vi "Compensate direction motor.vi"() -> ()   [LabVIEW 2011]
panel:
  out "DSO1072B":refnum<visa-resource-name>="USB0::0x0957::0x0588::CN55040431::INSTR"
  out "MUX RELAY":refnum<visa-resource-name>
  out "PWIDTH":dbl format="%#_6f"
  out "MAX AMP":dbl format="%#_6f"
  out "read buffer":string
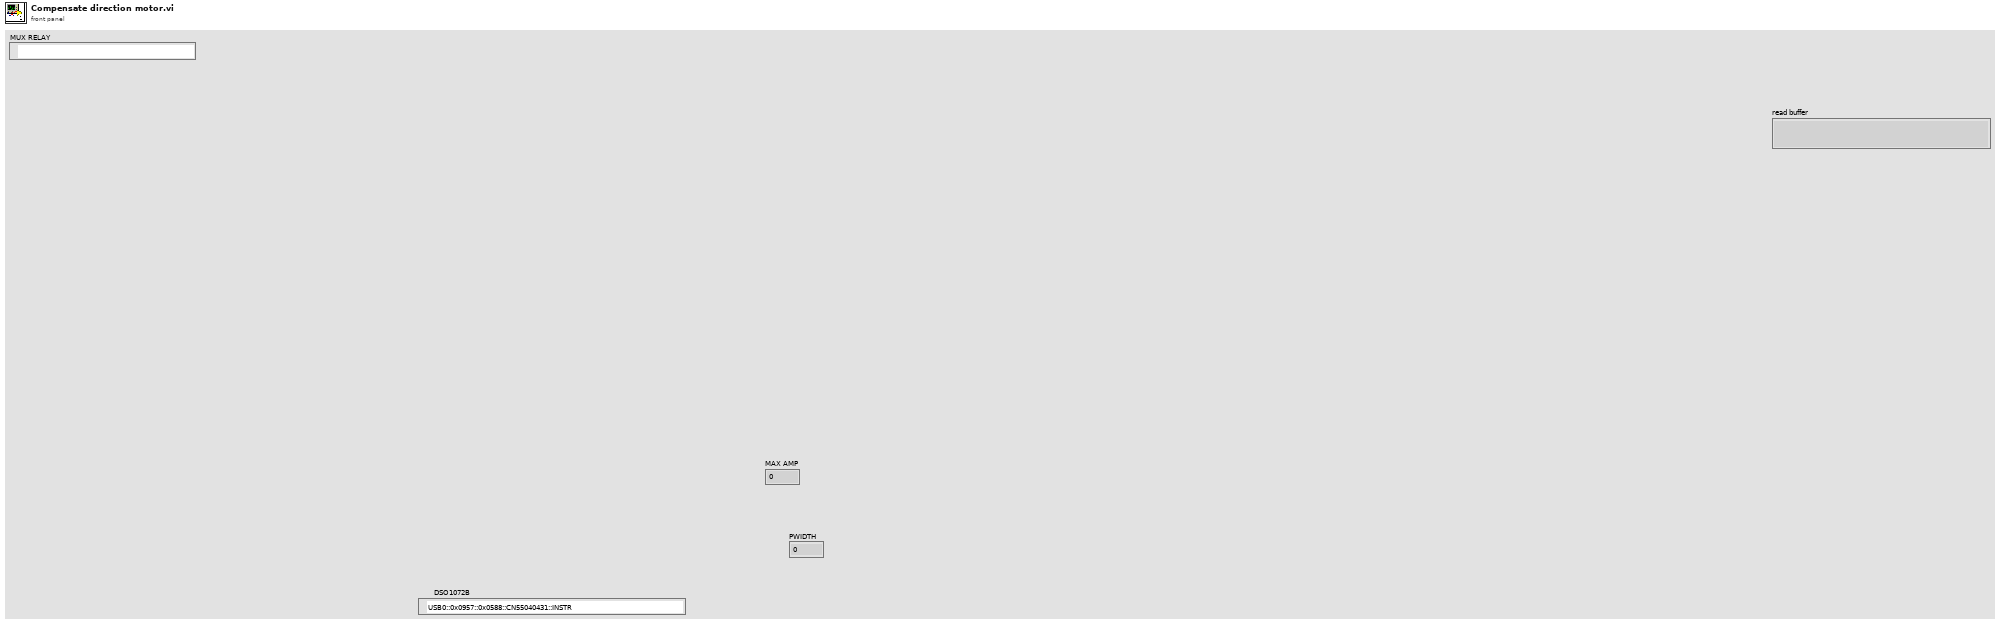
[diagram p1: front panel]
types:
  T1 = enum32{"Set Relay", "Append Relay", "Clear Relay", "Manual Cmd"}
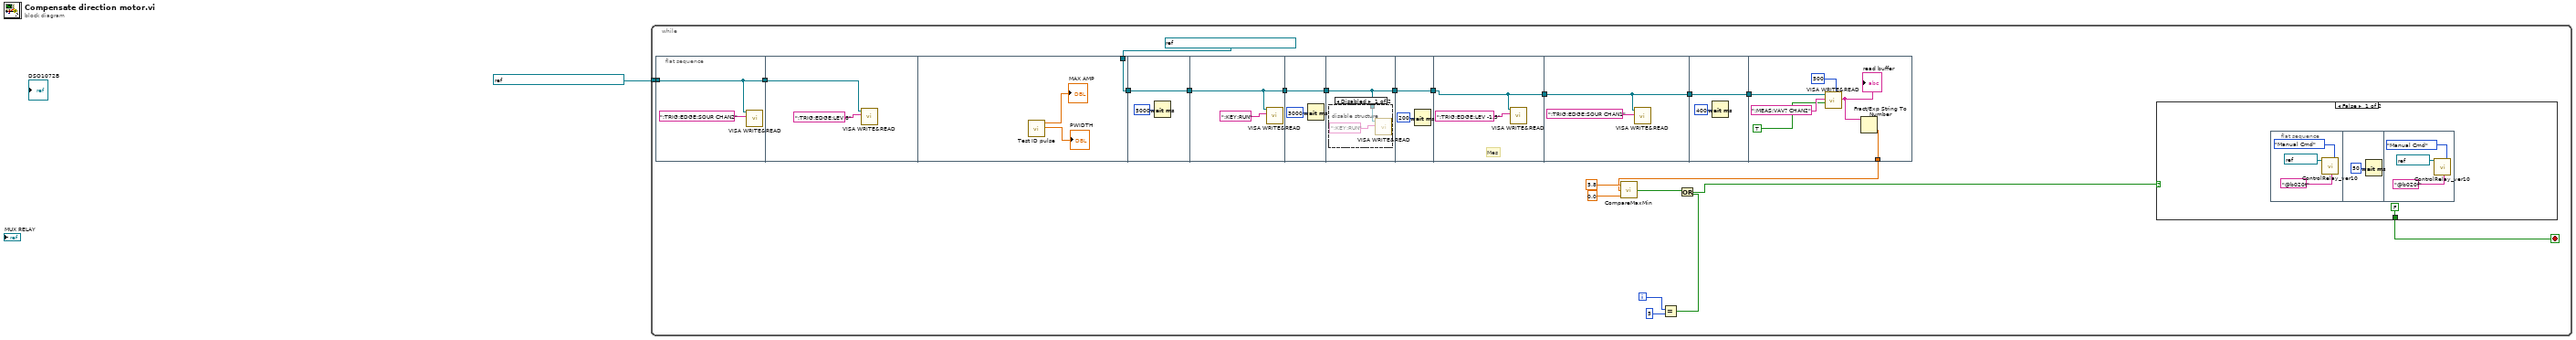
[diagram p0: block diagram]
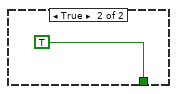
[diagram p2: hidden frame]
diagram:
  n1 = while {
    tunnel: refnum<visa-resource-name> "USB0::0x0957::0x0588::CN55433886::INSTR" ("VISA resource name In") -> [w10]
    i -> [w20]
    stop <- w15 stop-if-true
    n2 = flat-sequence {
      tunnel: w10 -> [w32]
      tunnel: [w32] -> w3
      tunnel: w3 -> [w34]
      tunnel: [w38] -> w14
      tunnel: refnum<visa-resource-name> "USB0::0x0957::0x0588::CN55433886::INSTR" ("VISA resource name In") -> [w38]
      tunnel: w14 -> [w39]
      tunnel: [w39] -> w11
      tunnel: w11 -> [w41]
      tunnel: [w41] -> w8
      tunnel: w8 -> [w44]
      tunnel: [w44] -> w7
      tunnel: w7 -> [w45]
      tunnel: [w45] -> w2
      tunnel: [w48] -> w4
      tunnel: w2 -> [w48]
      tunnel: w4 -> [w50]
      tunnel: [w50] -> w6
      tunnel: w6 -> [w53]
      tunnel: [w53] -> w5
      tunnel: w5 -> [w54]
      tunnel: [w54] -> w13
      tunnel: w13 -> [w60]
      tunnel: [w56] -> w9
      frame #0 {
        n3 = call "VISA WRITE&READ.vi"("write buffer"=":TRIG:EDGE:SOUR CHAN2", "VISA resource name In"=w32) -> ()  [unwired: 7 in, 3 out]
      }
      frame #1 {
        n4 = call "VISA WRITE&READ.vi"("write buffer"=":TRIG:EDGE:LEV 8", "VISA resource name In"=w34) -> ()  [unwired: 7 in, 3 out]
      }
      frame #2 {
        n5 = call "Test ID pulse.vi"() -> ("PWIDTH"=→"PWIDTH":dbl, "MAX AMP"=→"MAX AMP":dbl)  [unwired: 10 in]
      }
      frame #3 {
        n6 = Wait (ms)(milliseconds to wait=u32 5000) -> ()  [unwired: 1 out]
      }
      frame #4 {
        n7 = call "VISA WRITE&READ.vi"("write buffer"=":KEY:RUN", "VISA resource name In"=w41) -> ()  [unwired: 7 in, 3 out]
      }
      frame #5 {
        n8 = Wait (ms)(milliseconds to wait=u32 3000) -> ()  [unwired: 1 out]
      }
      frame #6 {
        n9 = disable-structure shown="Disabled" {
          disable-tunnel: w45 -> [w46 _]
          frame Disabled {
            n10 = call "VISA WRITE&READ.vi"("write buffer"=":KEY:RUN", "VISA resource name In"=w46) -> ()  [unwired: 7 in, 3 out]
          }
          frame Enabled {
          }
        }
      }
      frame #7 {
        n11 = Wait (ms)(milliseconds to wait=u32 200) -> ()  [unwired: 1 out]
      }
      frame #8 {
        # "Mes"
        n12 = call "VISA WRITE&READ.vi"("write buffer"=":TRIG:EDGE:LEV -1.5", "VISA resource name In"=w50) -> ()  [unwired: 7 in, 3 out]
      }
      frame #9 {
        n13 = call "VISA WRITE&READ.vi"("write buffer"=":TRIG:EDGE:SOUR CHAN1", "VISA resource name In"=w53) -> ()  [unwired: 7 in, 3 out]
      }
      frame #10 {
        n14 = Wait (ms)(milliseconds to wait=u32 400) -> ()  [unwired: 1 out]
      }
      frame #11 {
        n15 = call "VISA WRITE&READ.vi"("byte count"=u32 500, "Read?"=TRUE, "write buffer"=":MEAS:VAV? CHAN2", "VISA resource name In"=w60) -> ("read buffer"=w57:string)  [unwired: 5 in, 2 out]
        "read buffer" <- w57
        n16 = Fract/Exp String To Number(string=w57) -> (number=w56:dbl)  [unwired: 3 in, 1 out]
      }
    }
    n17 = call "CompareMaxMin.vi"("Min"=0.0, "X"=w9, "Max"=5.8) -> ("OutCompare"=w22:bool)
    n18 = Equal?(x=w20, y=5) -> (x = y?=w21:bool)
    n19 = Or(x=w22, y=w21) -> (x .or. y?=w16:bool)
    n20 = case shown="False" w16 {
      tunnel: [FALSE TRUE] -> w15
      frame False {
        n21 = flat-sequence {
          frame #0 {
            n22 = call "ControlRelay_ver10.vi"("VISA session"=refnum<visa-resource-name> "COM3", "write buffer"="@b020t", "Relay Setting"=T1."Manual Cmd") -> ()  [unwired: 13 in, 4 out]
          }
          frame #1 {
            n23 = Wait (ms)(milliseconds to wait=u32 50) -> ()  [unwired: 1 out]
          }
          frame #2 {
            n24 = call "ControlRelay_ver10.vi"("VISA session"=refnum<visa-resource-name> "COM3", "write buffer"="@b020f", "Relay Setting"=T1."Manual Cmd") -> ()  [unwired: 13 in, 4 out]
          }
        }
      }
      frame True {
      }
    }
  }
